vi "Automotive ECU - Shifter.vi"() -> ()   [LabVIEW 2013]
doc: "Sample numeric display item."
uses:
  <vilib>/NI Veristand/Display Template Support/Display Template Support.llb/cluster_Screen Item Settings.ctl
  <vilib>/NI Veristand/Display Template Support/Display Template Support.llb/cluster_Graph Scale Settings.ctl
  <vilib>/NI Veristand/Display Template Support/Display Template Support.llb/cluster_Graph Plot Settings.ctl
  NationalInstruments.VeriStand.SystemStorage
  <vilib>/NI Veristand/Display Template Support/Display Template Support.llb/enum_Display Template Handler Minimal To Widget Msg.ctl
  <vilib>/NI Veristand/Display Template Support/Display Template Support.llb/enum_Display Template Handler Minimal To Workspace.ctl
  Support/FNR Object Parameters.ctl
  Support/PWM Object Parameters.ctl
  <vilib>/NI Veristand/Execution/Workspace/NI VeriStand - Get Single Channel Value.vi
  <vilib>/NI Veristand/Execution/Workspace/NI_VS Workspace ExecutionAPI.lvlib
panel:
  in  "Shifter":enum32{"P", "R", "N"}(radio)=enum."R"
  in  "NIVS.System Definition Root":refnum<k24>
  in  "NIVS.Gateway IP Address":string
  out "Label":string="Numeric"
  in  "Item.Data":T1
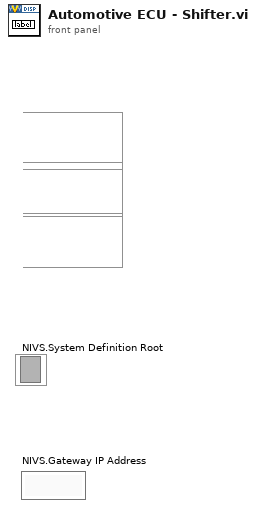
[diagram p1: front panel]
types:
  T1 = typedef "cluster_Screen Item Settings.ctl" = cluster{"Template VI":string, "Position X":i32, "Position Y":i32, "Custom":string, "Show Title Bar":bool, "ID":i32, "Always On Top":bool, "Allow Resize":bool, "Allow Minimize":bool, "Allow Close":bool, "Size to Screen":bool, "Screen.ID":i32, "State":enum16{"Normal", "New"}, "Title":string, "Window Bounds":cluster{"[0]":i16, "[1]":i16, "[2]":i16, "[3]":i16}, "Channel Ref":u64, "Unit":string, "Default Units?":bool, "Flash Limit?":bool, "Color 1":u32, "Color 2":u32, "Color 3":u32, "Color 4":u32, "Bck Color":u32, "Fore Color":u32, "Limit 1":dbl, "Limit 2":dbl, "Limit 3":dbl, "Limit 4":dbl, "Limit Mode 1":i32, "Limit Mode 2":i32, "Limit Mode 3":i32, "Limit Mode 4":i32, "Scale Precision":i32, "Scale Min":dbl, "Scale Max":dbl, "Format":i32, "Precision":i32, "Background Type":i32, "IDs":i32[], "Units":string[], "Labels":string[], "Scale Factor":dbl, "Scale Offset":dbl, "YScale Index":u32[], "XScale":T2, "YScales":T2[], "Plots":T3[], "Update Period":dbl, "History Length":dbl, "My.Ref":refnum<vi>, "Is Control?":bool, "Channel Paths":string[], "Custom Data":variant}
  T2 = typedef "cluster_Graph Scale Settings.ctl" = cluster{"Format":u8, "Precision":u8, "Fit":u8, "Label":string, "Use Default Label":bool, "Label Visible":bool, "Min":dbl, "Max":dbl}
  T3 = typedef "cluster_Graph Plot Settings.ctl" = cluster{"Bar Style":u8, "Fill To":i16, "Fill/PtColor":u32, "Line Style":u8, "Line Width":u8, "Color":u32, "Interp":u8, "Point Style":u8}
  T4 = typedef "enum_Display Template Handler Minimal To Workspace.ctl" = cluster{"Operation":enum16{"SetCustomData", "DeleteItem"}, "Data":variant}
  T5 = typedef "enum_Display Template Handler Minimal To Widget Msg.ctl" = enum16{"Stop", "LaunchConfigDialog"}
  T6 = typedef "FNR Object Parameters.ctl" = cluster{"PWM Config":T7, "PWM Settings":dbl[], "BG color":u32, "Obj Color":u32, "Initialized?":bool, "Default Control Values":variant[]}
  T7 = typedef "PWM Object Parameters.ctl" = cluster{"RIO?":bool, "Label":string, "PWM Channel Path":cluster{"NodePathArray":string[], "Node Path":string}}
  T8 = typedef "NI_VS Workspace ExecutionAPI.lvlib/WorkspaceAPI.ctl" = refnum<k24>
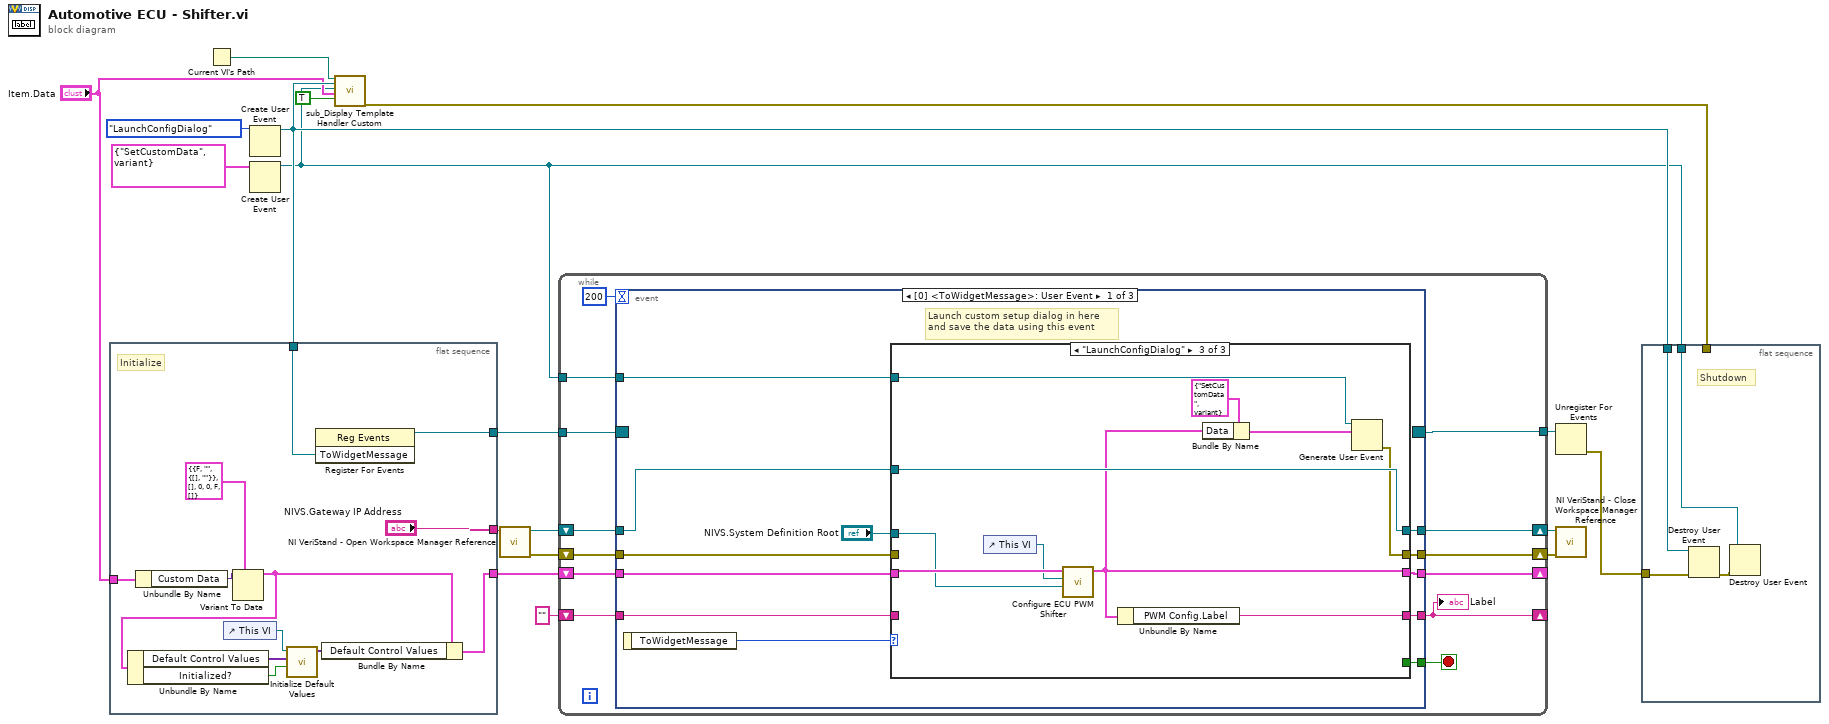
[diagram p0: block diagram]
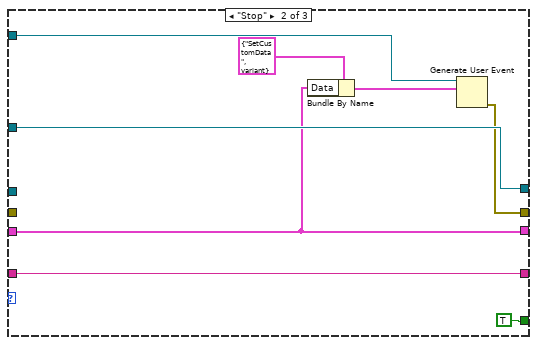
[diagram p3: hidden frame]
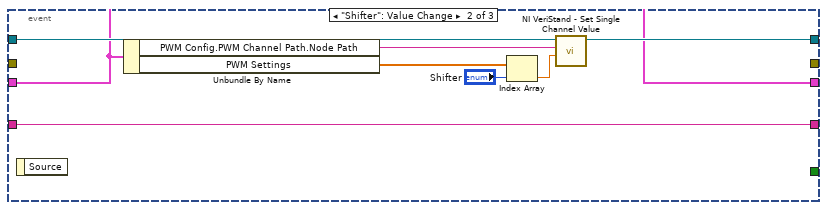
[diagram p4: hidden frame]
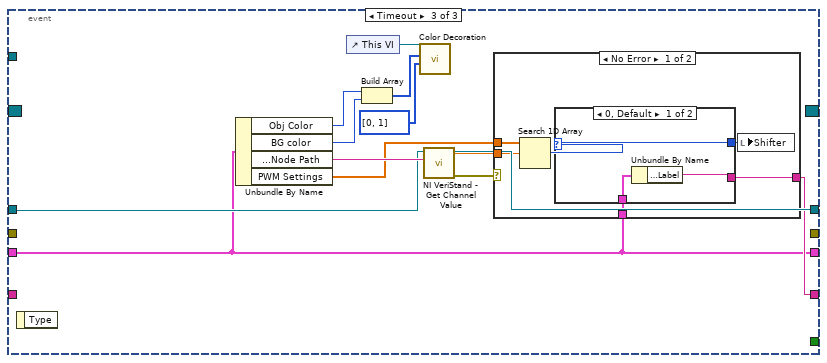
[diagram p5: hidden frame]
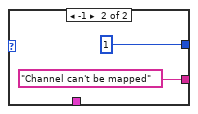
[diagram p6: hidden frame]
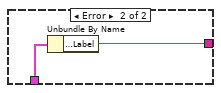
[diagram p7: hidden frame]
diagram:
  n1 = flat-sequence {
    tunnel: [w30] -> w16
    tunnel: w13 -> [w29]
    tunnel: "Item.Data" -> [w28]
    tunnel: [w19] -> w7
    tunnel: ["NIVS.Gateway IP Address"] -> w2
    frame #0 {
      # "Initialize"
      n2 = Unbundle By Name(w28) -> ("Custom Data"=w27:variant)
      n3 = control-ref of="This VI"() -> (w22:refnum<vi>)
      n4 = Variant To Data(type=T6 {"PWM Config"={"RIO?"=FALSE, "Label"="", "PWM Channel Path"={"NodePathArray"=[], "Node Path"=""}}, "PWM Settings"=[], "BG color"=0, "Obj Color"=0, "Initialized?"=FALSE, "Default Control Values"=[]} ("Cluster"), Variant=w27) -> (data=w20:T6)  [unwired: 1 in, 1 out]
      n5 = Unbundle By Name(w20) -> ("Default Control Values"=w23:variant[], "Initialized?"=w21:bool)
      n6 = call "Initialize Default Values.vi"("Initialized?"=w21, "Default Control Values in"=w23, "VI in"=w22) -> ("Default Control Values out"=w24:variant[])  [unwired: 7 in, 1 out]
      n7 = register-events(w29) -> (reference out=w30:refnum<event-registration>)  [unwired: 2 in, 1 out]
      n8 = Bundle By Name(cluster=w20, "Default Control Values"=w24) -> (w19:T6)
    }
  }
  n9 = Current VI's Path() -> (path=w11:path)
  n10 = Create User Event(user event datatype=enum_Display_Template_Handler_Minimal_To_Widget_Msg."LaunchConfigDialog" ("ToWidgetMessage")) -> (user event=w13:refnum<user-event>)  [unwired: 1 in, 1 out]
  n11 = Create User Event(user event datatype=T4 {"Operation"=enum."SetCustomData", "Data"=variant} ("Data")) -> (user event=w9:refnum<user-event>)  [unwired: 1 in, 1 out]
  n12 = call <vilib>:"sub_Display Template Handler Custom.vi"("Parent.Path"=w11, "ToWidgetEvent"=w13, "ToWorkspace"=w9, "Item.Data"="Item.Data", "Resizable"=TRUE) -> ("error out"=w18:errorcluster)  [unwired: 14 in]
  n13 = call <vilib>:"NI VeriStand - Open Workspace Manager Reference.vi"("Gateway IP Address (\"\": localhost)"=w2) -> ("error out"=w5:errorcluster, "WorkspaceManager"=w6:T8)  [unwired: 9 in]
  n14 = while {
    tunnel: w16 -> [w43]
    tunnel: [w41] -> w15
    tunnel: w9 -> [w40]
    shift-right: [w32] -> _
    shift-left: w7 -> [w39]
    shift-right: [w36] -> w4
    shift-left: w6 -> [w38]
    shift-right: [w33] -> w3
    shift-left: w5 -> [w37]
    shift-right: [w34] -> _
    shift-left: "" ("Out") -> [w35]
    stop <- w42 stop-if-true
    n15 = event shown="[0] <ToWidgetMessage>: User Event" {
      selector: w43 -> [_ _ _]
      dyn-events: [_ _ _] -> w41
      timeout: 200 -> [_ _ _]
      tunnel: [w54 _ _] -> w42
      tunnel: w40 -> [w53 _ _]
      tunnel: w39 -> [w49 w79 w87]
      tunnel: w38 -> [w52 w84 w92]
      tunnel: w37 -> [w47 _ _]
      tunnel: [w51 w81 w89] -> w36
      tunnel: [w46 _ _] -> w33
      tunnel: [w45 w80 w88] -> w34
      tunnel: w35 -> [w44 w80 _]
      tunnel: [w48 w79 w87] -> w32
      event User Event {
        # "Launch custom setup dialog in here\nand save the data using this event"
        n16 = event-data() -> ("ToWidgetMessage"=w55:T5)  [unwired: 1 out]
        n17 = case shown="\"LaunchConfigDialog\"" w55 {
          tunnel: [_ TRUE _] -> w54
          tunnel: w53 -> [_ w63 w72]
          tunnel: w52 -> [w59 w66 w77]
          tunnel: [w59 w66 w77] -> w51
          tunnel: "NIVS.System Definition Root" -> [_ _ w75]
          tunnel: w49 -> [w58 w62 w76]
          tunnel: [w58 w62 w71] -> w48
          tunnel: w47 -> [w56 _ _]
          tunnel: [w56 w61 w70] -> w46
          tunnel: [w57 w60 w69] -> w45
          tunnel: w44 -> [w57 w60 _]
          frame Default {
          }
          frame "Stop" {
            n18 = Bundle By Name(cluster=T4 {"Operation"=enum."SetCustomData", "Data"=variant} ("event data"), "Data"=w62) -> (w64:T4)
            n19 = Generate User Event(user event=w63, event data cluster=w64) -> (error out=w61:errorcluster)  [unwired: 2 in, 1 out]
          }
          frame "LaunchConfigDialog" {
            n20 = control-ref of="This VI"() -> (w68:refnum<vi>)
            n21 = call "Configure ECU PWM Shifter.vi"("NIVS.System Definition Root"=w75, "VI Reference"=w68, "FNR Data in"=w76) -> ("FNR Data Out"=w71:T6)  [unwired: 7 in, 1 out]
            n22 = Unbundle By Name(w71) -> ("PWM Config.Label"=w69:string)
            n23 = Bundle By Name(cluster=T4 {"Operation"=enum."SetCustomData", "Data"=variant} ("event data"), "Data"=w71) -> (w74:T4)
            n24 = Generate User Event(user event=w72, event data cluster=w74) -> (error out=w70:errorcluster)  [unwired: 2 in, 1 out]
          }
        }
      }
      event "Shifter": Value Change {
        n25 = event-data() -> ()  [unwired: 2 out]
        n26 = Unbundle By Name(w79) -> ("PWM Config.PWM Channel Path.Node Path"=w83:string, "PWM Settings"=w78:dbl[])
        n27 = Index Array(array=w78, index="Shifter") -> (element=w82:dbl)
        n28 = call <vilib>:"NI VeriStand - Set Single Channel Value.vi"("Value"=w82, "Channel"=w83, "WorkspaceManager in"=w84) -> ("WorkspaceManager out"=w81:T8)  [unwired: 7 in, 1 out]
      }
      event Timeout {
        n29 = event-data() -> ()  [unwired: 2 out]
        n30 = Unbundle By Name(w87) -> ("Obj Color"=w97:u32, "BG color"=w98:u32, "PWM Config.PWM Channel Path.Node Path"=w93:string, "PWM Settings"=w91:dbl[])
        n31 = control-ref of="This VI"() -> (w96:refnum<vi>)
        n32 = Build Array(w97, w98) -> (w94:u32[])
        n33 = call "Color Decoration.vi"("VI reference"=w96, "Color Array"=w94, "Index Array"=u32[] [0, 1]) -> ()  [unwired: 7 in, 1 out]
        n34 = call-poly <vilib>:"NI VeriStand - Get Channel Value.vi"("Channel"=w93, "WorkspaceManager in"=w92) -> ("error out"=w86:errorcluster, "Value"=w90:dbl, "WorkspaceManager out"=w89:T8)  [unwired: 7 in]
        n35 = case shown="No Error" w86 {
          tunnel: w91 -> [w104 _]
          tunnel: w90 -> [w103 _]
          tunnel: [w100 w110] -> w88
          tunnel: w87 -> [w99 w111]
          frame No Error {
            n36 = Search 1D Array(1D array=w104, element=w103) -> (index of element=w102:i32)  [unwired: 1 in]
            n37 = case shown="0, Default" w102 {
              selector: w102 -> [w107 _]
              tunnel: [w107 1 ("index of element")] -> w101
              tunnel: [w106 "Channel can't be mapped"] -> w100
              tunnel: w99 -> [w105 _]
              frame 0, Default {
                n38 = Unbundle By Name(w105) -> ("PWM Config.Label"=w106:string)
              }
              frame -1 {
              }
            }
            n39 = local write "Shifter"(w101) -> ()
          }
          frame Error {
            n40 = Unbundle By Name(w111) -> ("PWM Config.Label"=w110:string)
          }
        }
      }
    }
    "Label" <- w34
  }
  n41 = Unregister For Events(event registration refnum=w15) -> (error out=w14:errorcluster)  [unwired: 1 in]
  n42 = call <vilib>:"NI VeriStand - Close Workspace Manager Reference.vi"("error in (no error)"=w3, "WorkspaceManager"=w4) -> ()  [unwired: 9 in, 1 out]
  n43 = flat-sequence {
    tunnel: w18 -> [_]
    tunnel: w14 -> [w114]
    tunnel: w13 -> [w115]
    tunnel: w9 -> [w112]
    frame #0 {
      # "Shutdown"
      n44 = Destroy User Event(user event=w115, error in=w114) -> (error out=w113:errorcluster)
      n45 = Destroy User Event(user event=w112, error in=w113) -> ()  [unwired: 1 out]
    }
  }
